vi "operation.vi"(9 "Return Data (T)":bool=TRUE, 10 "Command Text":string) -> (3 "Data":string[][](array[string]))   [LabVIEW 2016, in "database.lvlib"]
uses:
  database.lvlib
panel:
  out "error create":errorcluster
  out "error open":errorcluster
  out "error out":errorcluster
  in  "error in (no error)":errorcluster
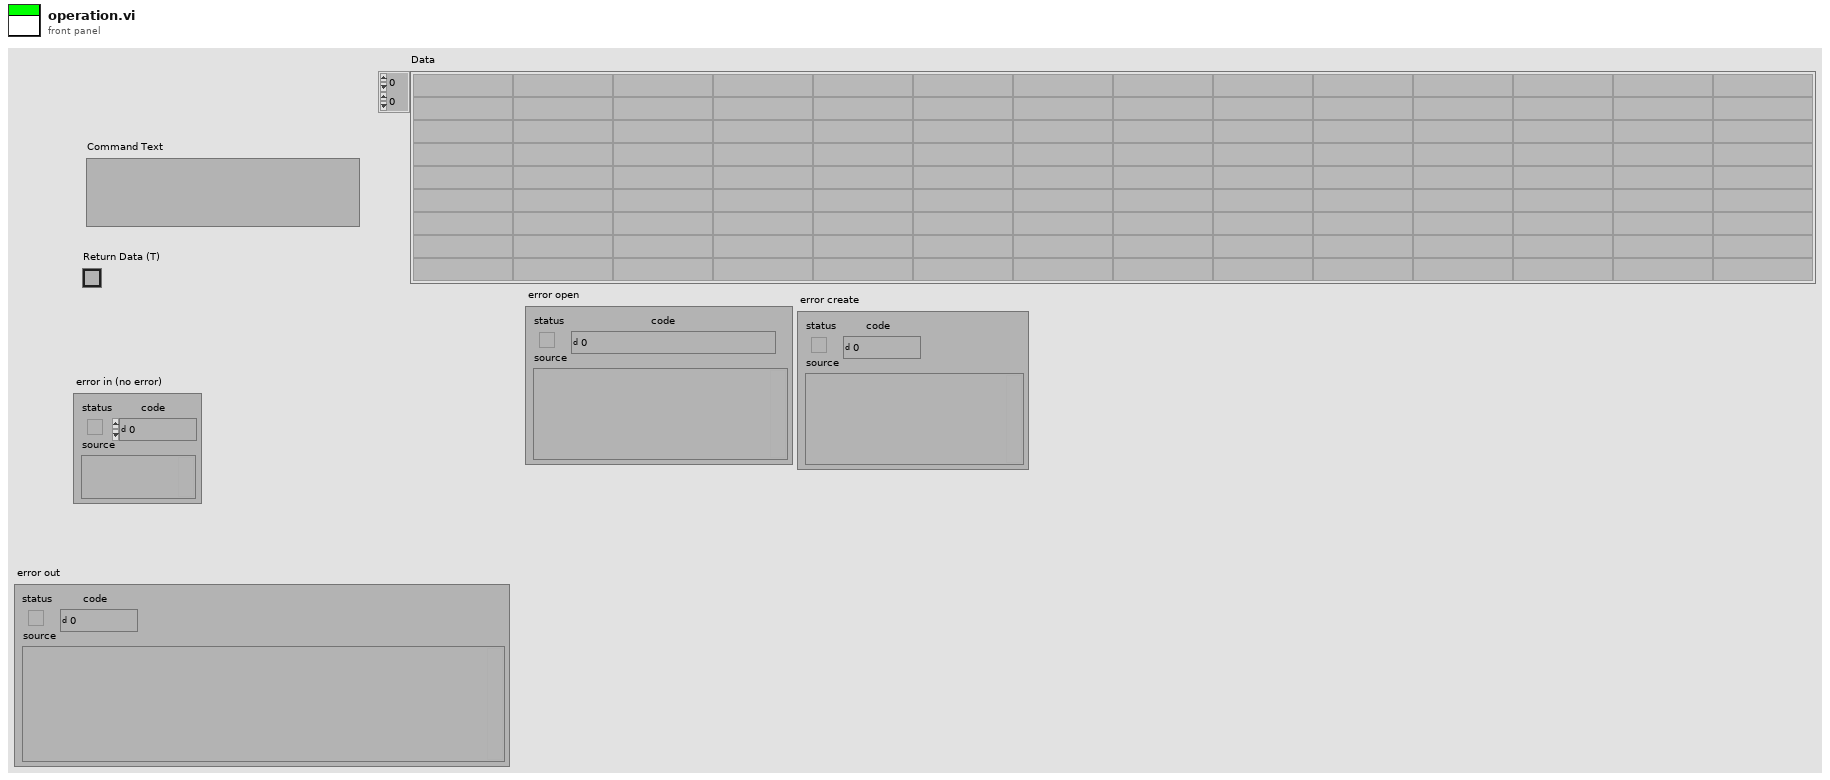
[diagram p1: front panel]
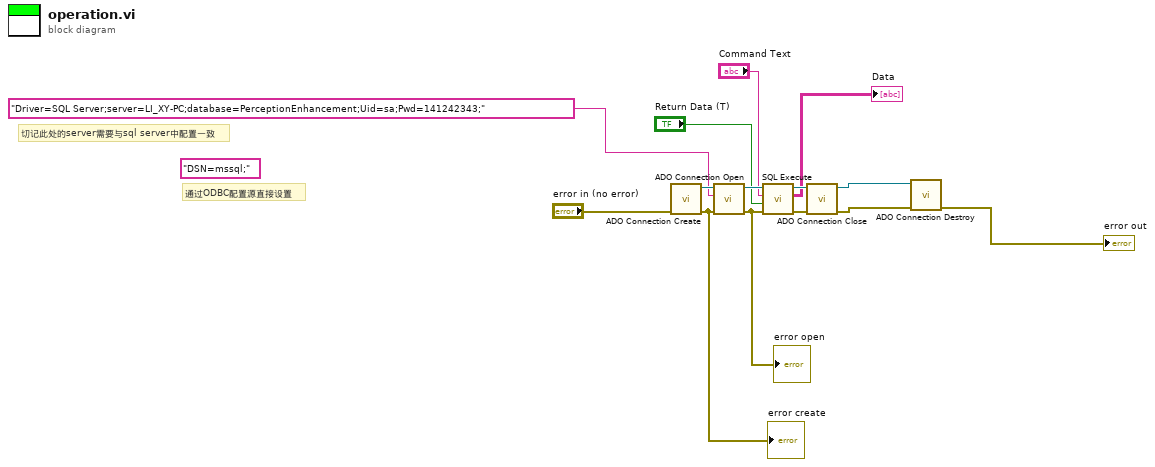
[diagram p0: block diagram]
diagram:
  (unwired) "DSN=mssql;" ("ConnectionString")
  # "切记此处的server需要与sql server中配置一致"
  # "通过ODBC配置源直接设置"
  n1 = call <userlib>:"ADO Connection Create.vi"("error in (no error)"="error in (no error)") -> ("error out"=w2:errorcluster, "ADODB._Connection Out"=w14:refnum<k7>)  [unwired: 9 in]
  "error create" <- w2
  n2 = call <userlib>:"ADO Connection Open.vi"("error in (no error)"=w2, "ConnectionString"="Driver=SQL Server;server=LI_XY-PC;database=PerceptionEnhancement;Uid=sa;Pwd=141242343;", "ADODB._Connection In"=w14) -> ("error out"=w12:errorcluster, "ADODB._Connection Out"=w13:refnum<k7>)  [unwired: 7 in]
  "error open" <- w12
  n3 = call <userlib>:"SQL Execute.vi"("error in (no error)"=w12, "Return Data (T)"="Return Data (T)", "Command Text"="Command Text", "ADODB._Connection In"=w13) -> ("error out"=w10:errorcluster, "Data"=→"Data":string[][], "ADODB._Connection Out"=w11:refnum<k7>)  [unwired: 4 in, 1 out]
  n4 = call <userlib>:"ADO Connection Close.vi"("error in (no error)"=w10, "ADODB._Connection In"=w11) -> ("error out"=w8:errorcluster, "ADODB._Connection Out"=w9:refnum<k7>)  [unwired: 8 in]
  n5 = call <userlib>:"ADO Connection Destroy.vi"("error in (no error)"=w8, "ADODB._Connection In"=w9) -> ("error out"=→"error out":errorcluster)  [unwired: 9 in]
